vi "TestGetOSPrimaryLanguage.vi"(8 "error in (no error)":errorcluster) -> (0 "error out":errorcluster)   [LabVIEW 2017]
uses:
  <vilib>/addons/_JKI Toolkits/Caraya/classes/Test/Test.lvclass
  <vilib>/addons/_JKI Toolkits/Caraya/classes/Assert/Assert.lvclass
  src/API/JKI Simple Localization.lvlib
panel:
  # "See block diagram for unit tests of Get OS Primary Language.vi"
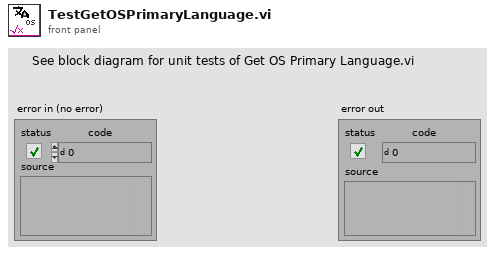
[diagram p1: front panel]
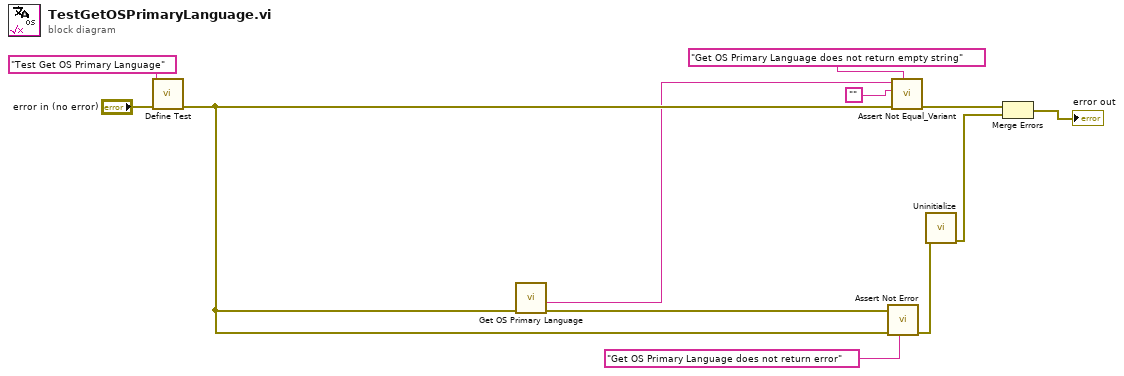
[diagram p0: block diagram]
diagram:
  n1 = call <vilib>:"Define Test.vi"("error in (no error)"="error in (no error)", "Label (VI Title)"="Test Get OS Primary Language") -> ("error out"=w4:errorcluster)  [unwired: 9 in]
  n2 = call "Get OS Primary Language.vi"("error in"=w4) -> ("error out"=w2:errorcluster, "OS Primary Language"=w3:string)  [unwired: 9 in]
  n3 = call <vilib>:"Assert Not Error.vi"("Label"="Get OS Primary Language does not return error", "error in (no error)"=w4, "Not Error?"=w2) -> ("error out"=w6:errorcluster)  [unwired: 8 in]
  n4 = call <vilib>:"Assert Not Equal_Variant.vi"("Label"="Get OS Primary Language does not return empty string", "error in (no error)"=w4, "Y"="", "X"=w3) -> ("error out"=w9:errorcluster)  [unwired: 7 in]
  n5 = call "Uninitialize.vi"("error in"=w6) -> ("error out"=w5:errorcluster)  [unwired: 10 in]
  n6 = Merge Errors(w9, w5) -> (→"error out":errorcluster)
